vi "Weighted Array RMS.vi"(8 "Error In":errorcluster, 9 "Weight Array":dbl[](array[numeric]), 11 "X Array":dbl[](array[numeric])) -> (0 "Error Out":errorcluster, 1 "Weighted":bool, 3 "RMS":dbl)   [LabVIEW 2021, in "Math.lvlib"]
uses:
  Math.lvlib
panel:
  # "see the License on the block diagram (Ctrl+E or Window:Show Block Diagram)"
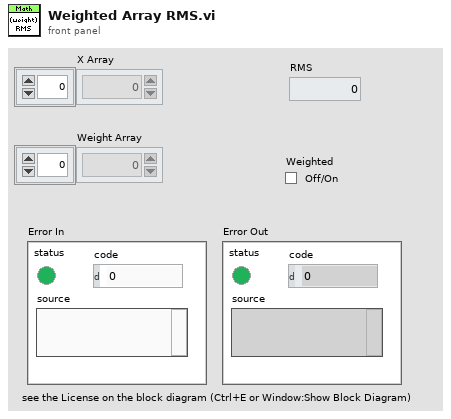
[diagram p1: front panel]
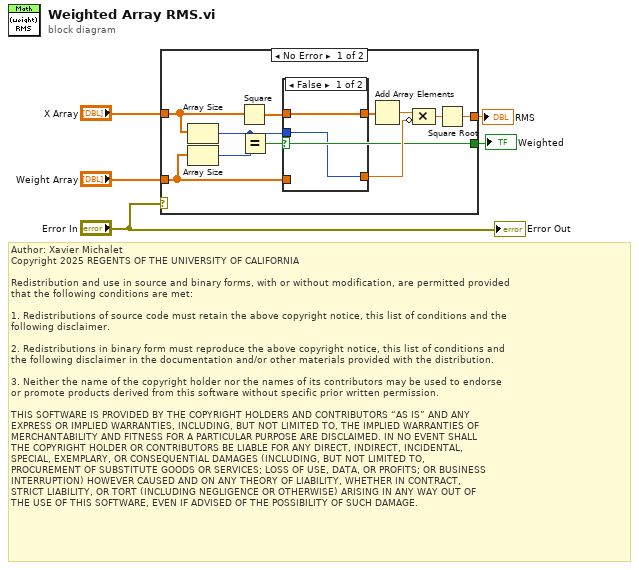
[diagram p0: block diagram]
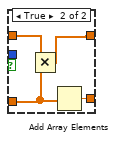
[diagram p2: hidden frame]
diagram:
  # "Author: Xavier Michalet\nCopyright 2025 REGENTS OF THE UNIVERSITY OF CALIFORNIA\n\nRedistribution and use in source and binary forms, with or without modification, are permitted provided\nthat the following conditions are met:\n\n1. Redistributions of source code must retain the above copyright notice, this list of conditions and the\nfollowing disclaimer.\n\n2. Redistributions in binary form must reproduce the above copyright notice, this list of conditions and\nthe following disclaimer in the documentation and/or other materials provided with the distribution.\n\n3. Neither the name of the copyright holder nor the names of its contributors may be used to endorse \nor promote products derived from this software without specific prior written permission.\n\nTHIS SOFTWARE IS PROVIDED BY THE COPYRIGHT HOLDERS AND CONTRIBUTORS “AS IS” AND ANY \nEXPRESS OR IMPLIED WARRANTIES, INCLUDING, BUT NOT LIMITED TO, THE IMPLIED WARRANTIES OF\nMERCHANTABILITY AND FITNESS FOR A PARTICULAR PURPOSE ARE DISCLAIMED. IN NO EVENT SHALL\nTHE COPYRIGHT HOLDER OR CONTRIBUTORS BE LIABLE FOR ANY DIRECT, INDIRECT, INCIDENTAL, \nSPECIAL, EXEMPLARY, OR CONSEQUENTIAL DAMAGES (INCLUDING, BUT NOT LIMITED TO, \nPROCUREMENT OF SUBSTITUTE GOODS OR SERVICES; LOSS OF USE, DATA, OR PROFITS; OR BUSINESS\nINTERRUPTION) HOWEVER CAUSED AND ON ANY THEORY OF LIABILITY, WHETHER IN CONTRACT, \nSTRICT LIABILITY, OR TORT (INCLUDING NEGLIGENCE OR OTHERWISE) ARISING IN ANY WAY OUT OF\nTHE USE OF THIS SOFTWARE, EVEN IF ADVISED OF THE POSSIBILITY OF SUCH DAMAGE."
  n1 = case shown="No Error" "Error In" {
    tunnel: "X Array" -> [w15 _]
    tunnel: "Weight Array" -> [w13 _]
    tunnel: [w7 _] -> w3
    tunnel: [w6 _] -> w1
    frame No Error {
      n2 = Array Size(array=w15) -> (size(s)=w9:i32)
      n3 = Array Size(array=w13) -> (size(s)=w16:i32)
      n4 = Square(x=w15) -> (x^2=w14:dbl[])
      n5 = Equal?(x=w9, y=w16) -> (x = y?=w6:bool)
      n6 = case shown="False" w6 {
        tunnel: w14 -> [w18 w22]
        tunnel: w13 -> [_ w20]
        tunnel: [w18 w21] -> w12
        tunnel: [w17 w19] -> w10
        tunnel: w9 -> [w17 _]
        frame False {
        }
        frame True {
          n7 = Multiply(x=w22, y=w20) -> (x*y=w21:dbl[])
          n8 = Add Array Elements(numeric array=w20) -> (sum=w19:dbl)
        }
      }
      n9 = Add Array Elements(numeric array=w12) -> (sum=w11:dbl)
      n10 = Compound Arithmetic op=MULTIPLY(w11, invert w10) -> (w8:dbl)
      n11 = Square Root(x=w8) -> (sqrt(x)=w7:dbl)
    }
    frame Error {
    }
  }
  "RMS" <- w3
  "Weighted" <- w1
  "Error Out" <- "Error In"
